vi "Acquisition Message Loop.vi"(0 "Message Queues":T1, 5 "Data Notifier":refnum<notifier>, 7 "Queue A - Processing":refnum<queue>, 9 "Queue B -TDMS Raw":refnum<queue>, 11 "error in (no error)":errorcluster) -> (15 "error out":errorcluster)   [LabVIEW 2026, in "Acquisition.lvlib"]
doc: "Message loop for handling messages pertaining to the acquisition of data from the hardware."
uses:
  Acquisition.lvlib
  support/Architecture/Message Queue/All Message Queues.ctl
  support/Architecture/Message Queue/Message Cluster.ctl
  controls/UI/UUT Display Data.ctl
  controls/UI/Acq Settings.ctl
  Instrument Specifications Configuration.ctl
  Instrument Specifications Cluster Configuration.ctl
  controls/UI/Measurement Role.ctl
  controls/UI/Config Settings.ctl
  Acquisition Context.ctl
  controls/Controller/Stimulus Settings.ctl
  controls/Controller/Stimulus Outputs.ctl
  controls/Controller/Stimulus Output.ctl
  controls/Controller/Controller Core Data.ctl
  controls/UI/Units Enum.ctl
  controls/UI/Signal Enum.ctl
  controls/Controller/Stimulus Output Configuration.ctl
  controls/Controller/Stimulus Role.ctl
  Acquisition State.ctl
  Acquisition Payload.ctl
  support/Architecture/Message Queue/Enqueue Message (Single).vi
  <vilib>/Utility/error.llb/Error Cluster From Error Code.vi
  <vilib>/ErrorRing/Error Ring.xnode
  support/Architecture/Message Queue/Message Queue.lvlib
  Settings/Settings.lvlib
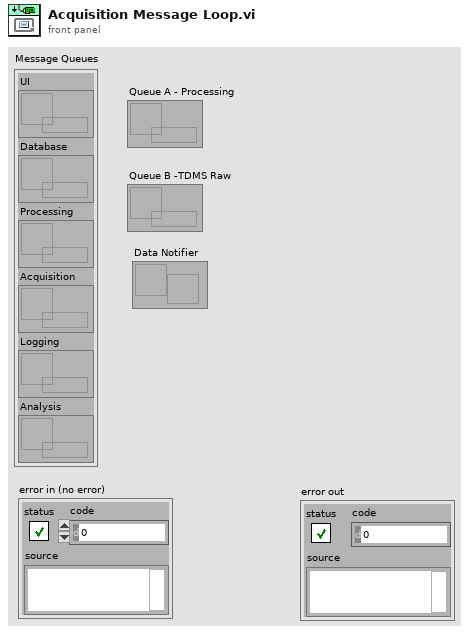
[diagram p1: front panel]
types:
  T1 = typedef "Message Queue.lvlib/All Message Queues.ctl" = cluster{"UI":refnum<queue>, "Database":refnum<queue>, "Processing":refnum<queue>, "Acquisition":refnum<queue>, "Logging":refnum<queue>, "Analysis":refnum<queue>}
  T2 = typedef "Settings.lvlib/Stimulus Settings.ctl" = cluster{"Stimulus Outputs":T3}
  T3 = typedef "Settings.lvlib/Stimulus Outputs.ctl" = T4[]
  T4 = typedef "Settings.lvlib/Stimulus Output.ctl" = cluster{"Controller Core Data":T5, "Stimulus Output Configuration":T8}
  T5 = typedef "Settings.lvlib/Controller Core Data.ctl" = cluster{"Min":dbl, "Max":dbl, "Units":T6, "Input Signal Type":T7, "Input Signal Min":dbl, "Input Signal Max":dbl}
  T6 = typedef "Units Enum.ctl" = enum16{"PSI", "Deg C", "kPa", "GPM"}
  T7 = typedef "Signal Enum.ctl" = enum16{"4-20mA", "0-10V", "Thermocouple Type K"}
  T8 = typedef "Settings.lvlib/Stimulus Output Configuration.ctl" = cluster{"DAQmx AO Physical Channel":tag, "Role":T9, "Model Numbers":string, "Serial Numbers":string, "Row":i32}
  T9 = typedef "Stimulus Role.ctl" = enum16{"Pressure Controller", "Temperature Controller"}
  T10 = typedef "Acquisition.lvlib/Acquisition Context.ctl" = cluster{"Setpoint":dbl, "Previous Setpoint":dbl, "Transition Start Time":dbl, "Transition Active?":bool, "Acknowledgement Pending?":bool}
  T11 = typedef "Acq Settings.ctl" = cluster{"Instrument Specifications":T12, "Config Settings":T15}
  T12 = typedef "Acquisition.lvlib/Instrument Specifications Configuration.ctl" = T13[]
  T13 = typedef "Acquisition.lvlib/Instrument Specifications Cluster Configuration.ctl" = cluster{"Sensor ID *":i32, "Target Sample Rate (Hz) *":dbl, "Steady-State Duration (s) *":i32, "Allowed Tolerance (%) FS *":dbl, "Max Settling Timeout (s) *":i32, "Physical Channel":string, "Measurement Role":T14}
  T14 = typedef "Settings.lvlib/Measurement Role.ctl" = enum16{"Controller", "Reference", "UUT", "Disable", "All"}
  T15 = typedef "Config Settings.ctl" = cluster{"Simulated Sensor Injection":dbl, "Base Device Name":string, "Simulation Mode":string}
  T16 = typedef "Acquisition.lvlib/Acquisition State.ctl" = enum16{"Idle", "Acquiring"}
  T17 = typedef "Acquisition.lvlib/Acquisition Payload.ctl" = cluster{"Acq Settings":T11, "Acquisition Context":T10, "Stimulus Settings":T2}
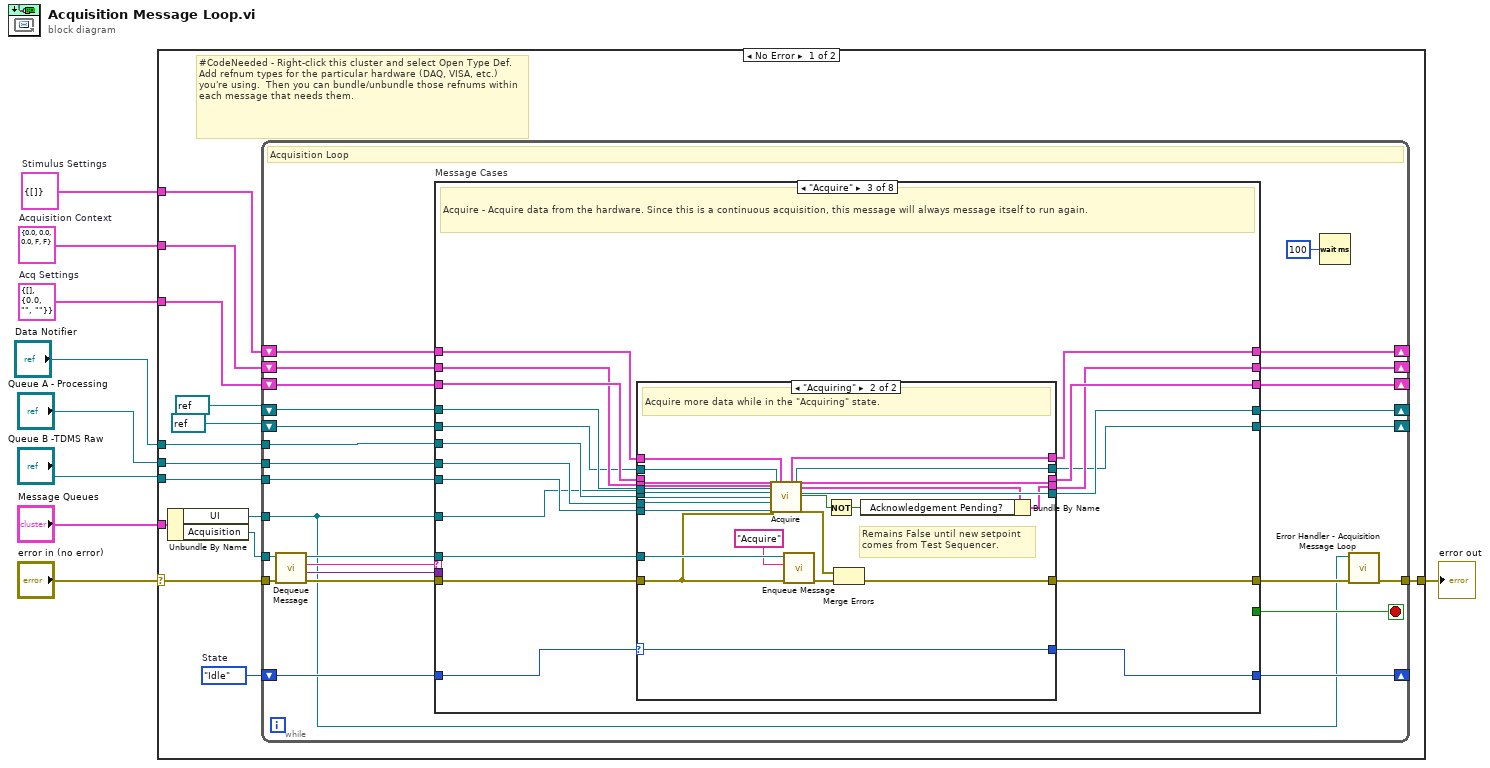
[diagram p0: block diagram]
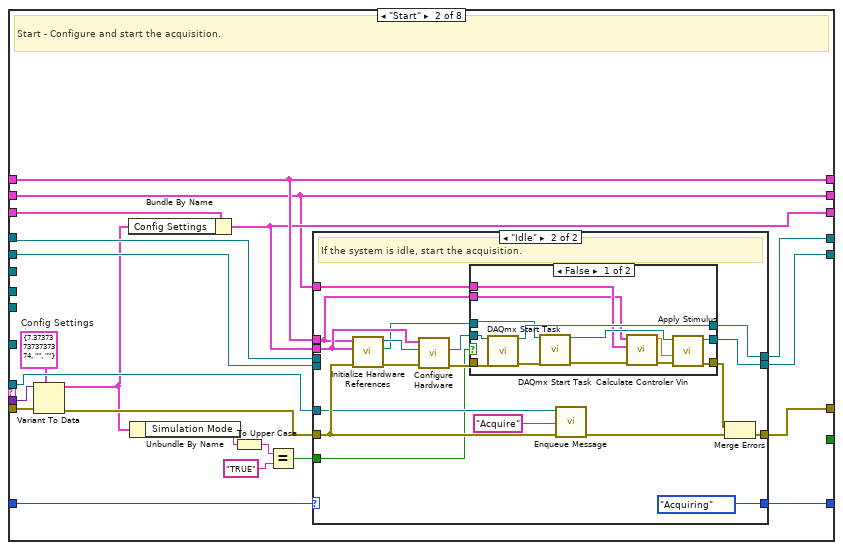
[diagram p3: hidden frame]
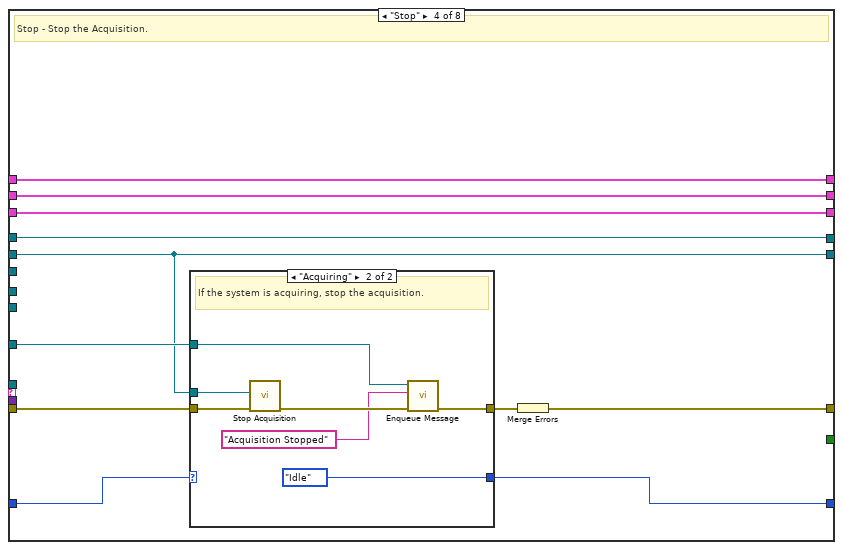
[diagram p7: hidden frame]
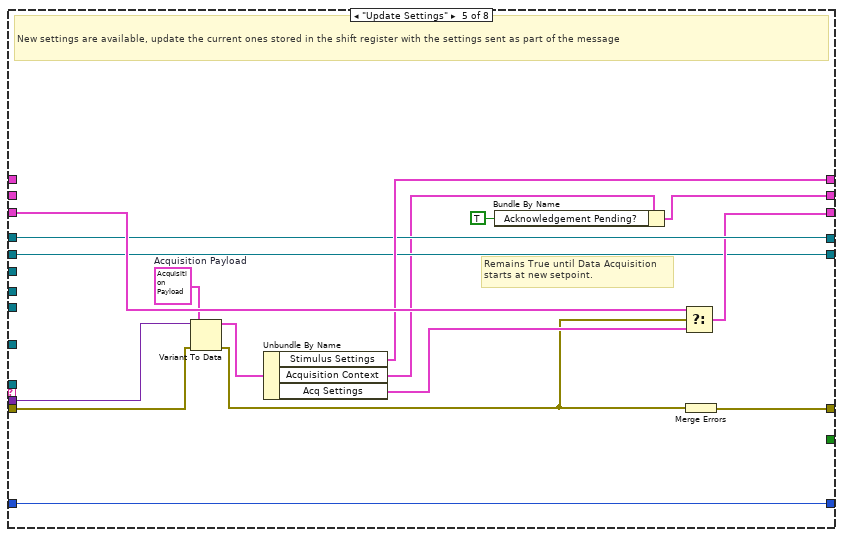
[diagram p9: hidden frame]
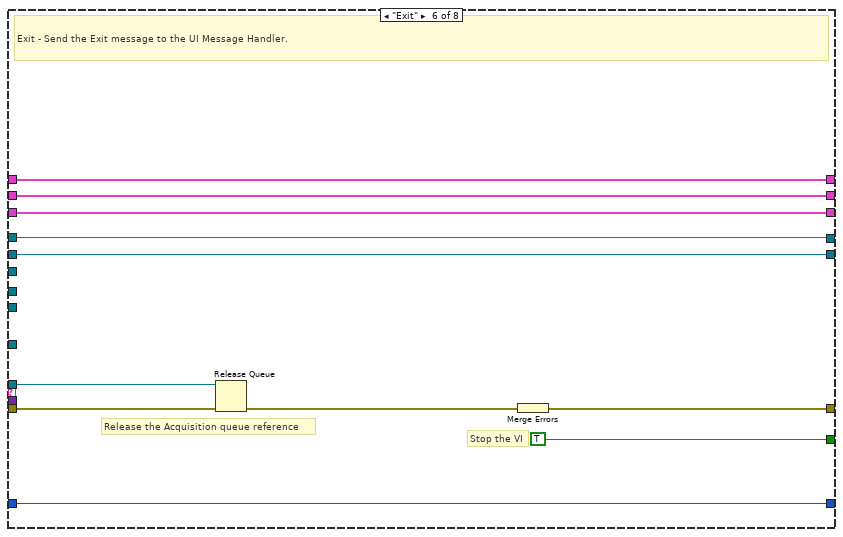
[diagram p10: hidden frame]
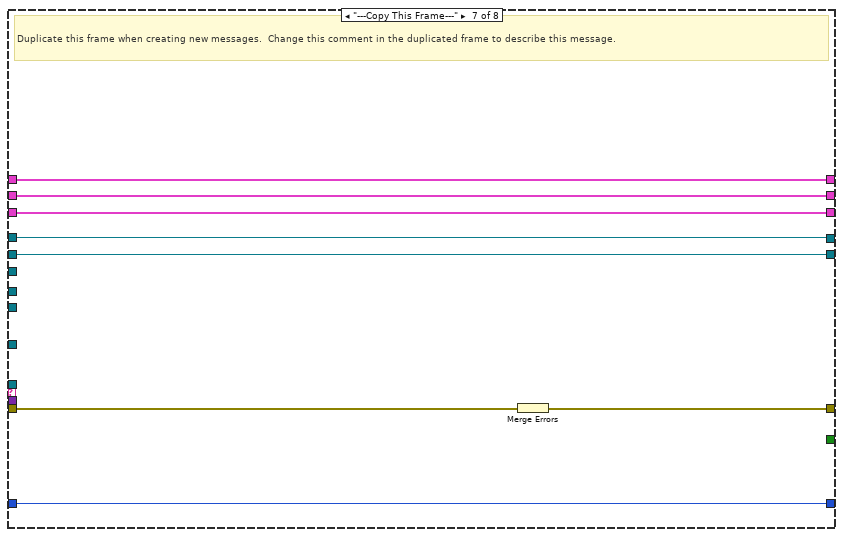
[diagram p11: hidden frame]
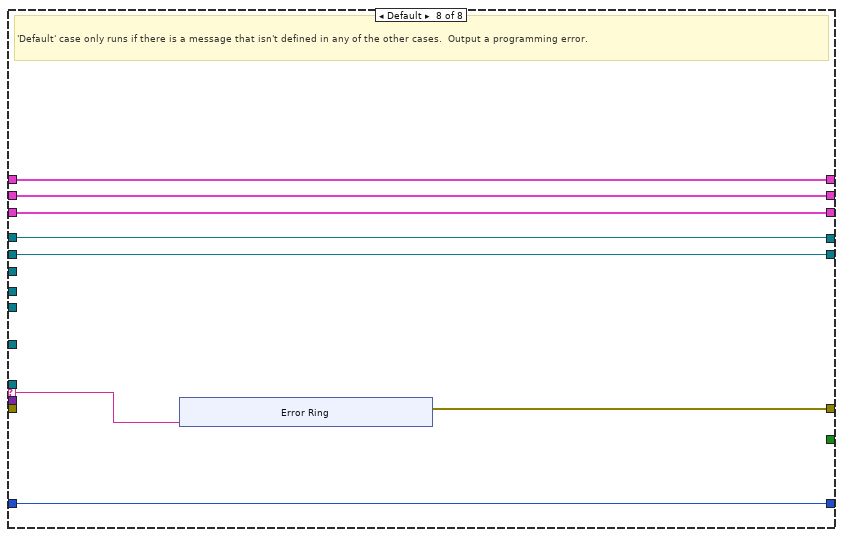
[diagram p12: hidden frame]
diagram:
  w2 = T2 {"Stimulus Outputs"=[]}  # Stimulus Settings
  w3 = T10 {"Setpoint"=0.0, "Previous Setpoint"=0.0, "Transition Start Time"=0.0, "Transition Active?"=FALSE, "Acknowledgement Pending?"=FALSE}  # Acquisition Context
  w4 = T11 {"Instrument Specifications"=[], "Config Settings"={"Simulated Sensor Injection"=0.0, "Base Device Name"="", "Simulation Mode"=""}}  # Acq Settings
  n1 = case shown="No Error" "error in (no error)" {
    selector: "error in (no error)" -> [w20 w236]
    tunnel: "Message Queues" -> [w23 _]
    tunnel: [w21 w236] -> w8
    tunnel: "Data Notifier" -> [w18 _]
    tunnel: "Queue B -TDMS Raw" -> [w17 _]
    tunnel: w4 -> [w15 _]
    tunnel: "Queue A - Processing" -> [w13 _]
    tunnel: w3 -> [w12 _]
    tunnel: w2 -> [w11 _]
    frame No Error {
      w16 = Acquisition_State."Idle"  # State
      # "#CodeNeeded - Right-click this cluster and select Open Type Def.  Add refnum types for the particular hardware (DAQ, VISA, etc.) you're using.  Then you can bundle/unbundle those refnums within each message that needs them."
      n2 = Unbundle By Name(w23) -> ("UI"=w19:refnum<queue>, "Acquisition"=w22:refnum<queue>)
      n3 = while {
        tunnel: w22 -> [w44]
        shift-right: [w26] -> _
        shift-left: w15 -> [w35]
        tunnel: w19 -> [w36]
        tunnel: w18 -> [w43]
        tunnel: w17 -> [w42]
        shift-right: [w40] -> _
        shift-left: w16 -> [w41]
        tunnel: w20 -> [w48]
        tunnel: [w39] -> w21
        shift-right: [w34] -> _
        shift-left: refnum<k21> refnum ("task out") -> [w33]
        tunnel: w13 -> [w32]
        shift-right: [w29] -> _
        shift-left: w12 -> [w30]
        shift-right: [w28] -> _
        shift-left: w11 -> [w27]
        shift-right: [w25] -> _
        shift-left: refnum<k21> refnum ("Calibration Task out") -> [w24]
        stop <- w49 stop-if-true
        # "Acquisition Loop"
        n4 = call "Dequeue Message.vi"("error in (no error)"=w48, "Message Queue"=w44) -> ("error out"=w47:errorcluster, "Message Data"=w45:variant, "Message"=w46:string, "dup Message Queue"=w37:refnum<queue>)  [unwired: 6 in]
        n5 = case "Message Cases" shown="\"Acquire\"" w46 {
          selector: w46 -> [_ _ _ _ _ _ _ w226]
          tunnel: w37 -> [_ w74 w133 _ _ w208 _ _]
          tunnel: w47 -> [w56 w73 w132 w175 w190 w210 w220 _]
          tunnel: [w56 w77 w134 w176 w201 w211 w219 w227] -> w38
          tunnel: [_ _ _ _ _ TRUE _ _] -> w49
          tunnel: w45 -> [_ w71 _ _ w200 _ _ _]
          tunnel: w36 -> [_ _ w120 w171 _ _ _ _]
          tunnel: w43 -> [_ _ w131 _ _ _ _ _]
          tunnel: w42 -> [_ _ w130 _ _ _ _ _]
          tunnel: w41 -> [w55 w75 w128 w173 w199 w207 w218 w228]
          tunnel: [w55 w76 w129 w172 w199 w207 w218 w228] -> w40
          tunnel: w35 -> [w51 w70 w126 w170 w198 w206 w217 w225]
          tunnel: [w54 w69 w118 w166 w191 w205 w216 w224] -> w34
          tunnel: w33 -> [w54 w68 w119 w166 w191 w205 w216 w224]
          tunnel: w32 -> [_ _ w127 _ _ _ _ _]
          tunnel: w30 -> [w53 w62 w125 w169 _ w204 w215 w223]
          tunnel: [w53 w62 w121 w169 w186 w204 w215 w223] -> w29
          tunnel: [w52 w66 w116 w168 w194 w203 w214 w222] -> w28
          tunnel: w27 -> [w52 w66 w117 w168 _ w203 w214 w222]
          tunnel: [w50 w65 w122 w167 w193 w202 w213 w221] -> w25
          tunnel: [w51 w64 w123 w170 w192 w206 w217 w225] -> w26
          tunnel: w24 -> [w50 w63 w124 w167 w193 w202 w213 w221]
          frame "Initialize" {
            # "Initialize  - Initialize is currently a no-op.  The hardware initialization takes place in the 'Start' message."
          }
          frame "Start" {
            w67 = T15 {"Simulated Sensor Injection"=7.373737373737374, "Base Device Name"="", "Simulation Mode"=""}  # Config Settings
            # "Start - Configure and start the acquisition."
            n6 = Variant To Data(error in=w73, type=w67, Variant=w71) -> (data=w58:T15, error out=w72:errorcluster)
            n7 = Bundle By Name(cluster=w70, "Config Settings"=w58) -> (w64:T11)
            n8 = Unbundle By Name(w58) -> ("Simulation Mode"=w61:string)
            n9 = To Upper Case(1:w61) -> (0:w60:string)
            n10 = Equal?(x=w60, y="TRUE") -> (x = y?=w57:bool)
            n11 = case shown="\"Idle\"" w75 {
              selector: w75 -> [w80 _]
              tunnel: [w81 w99] -> w77
              tunnel: w64 -> [_ w92]
              tunnel: w72 -> [w81 w98]
              tunnel: w74 -> [_ w96]
              tunnel: [w80 Acquisition_State."Acquiring" ("Acquisition State")] -> w76
              tunnel: [w79 w86] -> w69
              tunnel: w68 -> [w79 _]
              tunnel: w66 -> [_ w82]
              tunnel: [w78 w88] -> w65
              tunnel: w63 -> [w78 _]
              tunnel: w62 -> [_ w85]
              tunnel: w57 -> [_ w83]
              frame "Acquiring" {
                # "The system is already acquiring. Ignore the \"Start\" message."
              }
              frame "Idle" {
                # "If the system is idle, start the acquisition."
                n12 = call "Initialize Hardware References.vi"("error in (no error)"=w98, "Acq Settings in"=w92, "Stimulus Settings in"=w82) -> ("error out"=w95:errorcluster, "Stimulus Task"=w84:refnum<k21>, "Calibration Task"=w90:refnum<k21>)  [unwired: 4 in]
                n13 = call "Configure Hardware.vi"("error in (no error)"=w95, "Calibration Task in"=w90, "Acq Settings in"=w92) -> ("error out"=w91:errorcluster, "Calibration Task out"=w89:refnum<k21>)  [unwired: 6 in, 1 out]
                n14 = case shown="False" w83 {
                  tunnel: w91 -> [w112 w113]
                  tunnel: w89 -> [w111 w115]
                  tunnel: [w110 w115] -> w88
                  tunnel: [w109 w113] -> w87
                  tunnel: [w108 w114] -> w86
                  tunnel: w85 -> [w101 _]
                  tunnel: w84 -> [w103 w114]
                  tunnel: w82 -> [w100 _]
                  frame False {
                    n15 = call <vilib>:"DAQmx Start Task.vi"("task/channels in"=w111, "error in"=w112) -> ("task out"=w110:refnum<k21>, "error out"=w102:errorcluster)  [unwired: 12 in]
                    n16 = call <vilib>:"DAQmx Start Task.vi"("task/channels in"=w103, "error in"=w102) -> ("task out"=w104:refnum<k21>, "error out"=w107:errorcluster)  [unwired: 12 in]
                    n17 = call "Calculate Controler Vin.vi"("error in (no error)"=w107, "Acquisition Context"=w101, "Stimulus Settings"=w100) -> ("error out"=w106:errorcluster, "Vin"=w105:dbl)  [unwired: 7 in]
                    n18 = call "Apply Stimulus.vi"("error in (no error)"=w106, "Vin"=w105, "Stimulus Task in"=w104) -> ("error out"=w109:errorcluster, "Stimulus Task out"=w108:refnum<k21>)  [unwired: 7 in]
                  }
                  frame True {
                  }
                }
                n19 = call-poly "Enqueue Message.vi"("error in (no error)"=w98, "Message"="Acquire", "Message Queue"=w96) -> ("error out"=w97:errorcluster)  [unwired: 7 in, 1 out]
                n20 = Merge Errors(w87, w97) -> (w99:errorcluster)
              }
            }
          }
          frame "Acquire" {
            # "Acquire - Acquire data from the hardware. Since this is a continuous acquisition, this message will always message itself to run again."
            n21 = case shown="\"Acquiring\"" w128 {
              selector: w128 -> [w140 w159]
              tunnel: [w141 w165] -> w134
              tunnel: w133 -> [_ w163]
              tunnel: w132 -> [w141 w158]
              tunnel: w124 -> [w138 w153]
              tunnel: w131 -> [_ w154]
              tunnel: w130 -> [_ w160]
              tunnel: [w140 w159] -> w129
              tunnel: w127 -> [_ w155]
              tunnel: w126 -> [w139 w157]
              tunnel: [w139 w156] -> w123
              tunnel: w125 -> [w137 w152]
              tunnel: [w138 w151] -> w122
              tunnel: [w137 w149] -> w121
              tunnel: w120 -> [_ w146]
              tunnel: w119 -> [w136 w145]
              tunnel: [w136 w144] -> w118
              tunnel: w117 -> [w135 w143]
              tunnel: [w135 w142] -> w116
              frame "Idle" {
                # "Ignore \"Acquire\" messages when the acquisition is idle."
              }
              frame "Acquiring" {
                # "Remains False until new setpoint\ncomes from Test Sequencer."
                # "Acquire more data while in the \"Acquiring\" state."
                n22 = call "Acquire.vi"("Acq Settings in"=w157, "Acquisition Context in"=w152, "Calibration in"=w153, "UI"=w146, "Data Notifier"=w154, "Queue A - Processing"=w160, "Queue B -TDMS Raw"=w155, "error in (no error)"=w158, "Stimulus in"=w145, "Stimulus Settings in"=w143) -> ("Stimulus Settings out"=w142:T2, "Stimulus out"=w144:refnum<k21>, "Acq Settings out"=w156:T11, "Acquisition Context out"=w150:T10, "Calibration out"=w151:refnum<k21>, "Acknowledged?"=w147:bool, "error out"=w162:errorcluster)  [unwired: 11 in]
                n23 = call-poly "Enqueue Message.vi"("error in (no error)"=w158, "Message"="Acquire", "Message Queue"=w163) -> ("error out"=w164:errorcluster)  [unwired: 7 in, 1 out]
                n24 = Not(x=w147) -> (.not. x?=w148:bool)
                n25 = Merge Errors(w162, w164) -> (w165:errorcluster)
                n26 = Bundle By Name(cluster=w150, "Acknowledgement Pending?"=w148) -> (w149:T10)
              }
            }
          }
          frame "Stop" {
            # "Stop - Stop the Acquisition."
            n27 = case shown="\"Acquiring\"" w173 {
              selector: w173 -> [w177 _]
              tunnel: w175 -> [w178 w185]
              tunnel: [w178 w182] -> w174
              tunnel: [w177 Acquisition_State."Idle" ("State")] -> w172
              tunnel: w171 -> [_ w181]
              tunnel: w166 -> [_ w179]
              frame "Idle" {
                # "The system is already idle. Ignore the \"Stop\" message."
              }
              frame "Acquiring" {
                # "If the system is acquiring, stop the acquisition."
                n28 = call "Stop Acquisition.vi"("error in (no error)"=w185, "task in"=w179) -> ("error out"=w184:errorcluster)  [unwired: 9 in]
                n29 = call-poly "Enqueue Message.vi"("error in (no error)"=w184, "Message"="Acquisition Stopped", "Message Queue"=w181) -> ("error out"=w182:errorcluster)  [unwired: 7 in, 1 out]
              }
            }
            n30 = Merge Errors(w174) -> (w176:errorcluster)
          }
          frame "Update Settings" {
            w197 = T17 {"Acq Settings"={"Instrument Specifications"=[], "Config Settings"={"Simulated Sensor Injection"=0.0, "Base Device Name"="", "Simulation Mode"=""}}, "Acquisition Context"={"Setpoint"=0.0, "Previous Setpoint"=0.0, "Transition Start Time"=0.0, "Transition Active?"=FALSE, "Acknowledgement Pending?"=FALSE}, "Stimulus Settings"={"Stimulus Outputs"=[]}}  # Acquisition Payload
            # "Remains True until Data Acquisition\nstarts at new setpoint."
            # "New settings are available, update the current ones stored in the shift register with the settings sent as part of the message"
            n31 = Variant To Data(error in=w190, type=w197, Variant=w200) -> (data=w196:T17, error out=w189:errorcluster)
            n32 = Unbundle By Name(w196) -> ("Stimulus Settings"=w194:T2, "Acquisition Context"=w187:T10, "Acq Settings"=w195:T11)
            n33 = Bundle By Name(cluster=w187, "Acknowledgement Pending?"=TRUE) -> (w186:T10)
            n34 = Select(t=w198, s=w189, f=w195) -> (s? t:f=w192:T11)
            n35 = Merge Errors(w189) -> (w201:errorcluster)
          }
          frame "Exit" {
            # "Release the Acquisition queue reference"
            # "Stop the VI"
            # "Exit - Send the Exit message to the UI Message Handler."
            n36 = Release Queue(queue=w208, error in (no error)=w210) -> (error out=w209:errorcluster)  [unwired: 1 in, 2 out]
            n37 = Merge Errors(w209) -> (w211:errorcluster)
          }
          frame "---Copy This Frame---" {
            # "Duplicate this frame when creating new messages.  Change this comment in the duplicated frame to describe this message."
            n38 = Merge Errors(w220) -> (w219:errorcluster)
          }
          frame Default {
            # "'Default' case only runs if there is a message that isn't defined in any of the other cases.  Output a programming error."
            n39 = xnode "Error Ring"("parameter 0"=w226) -> ("error out"=w227:errorcluster)
          }
        }
        n40 = Wait (ms)(milliseconds to wait=u32 100) -> ()  [unwired: 1 out]
        n41 = call "Error Handler - Acquisition Message Loop.vi"("error in (no error)"=w38, "Message Queue"=w36) -> ("dup error in"=w39:errorcluster)  [unwired: 8 in, 1 out]
      }
    }
    frame Error {
    }
  }
  "error out" <- w8
